vi "Connect to Slave.vi"(8 "error in (no error)":errorcluster, 11 "TCP master in":refnum<class "TCP.lvclass">) -> (0 "error out":errorcluster, 3 "TCP master out":refnum<class "TCP.lvclass">)   [LabVIEW 2021, in "TCP.lvclass"]
doc: "Opens a TCP connection to the address and port stored in the class."
uses:
  TCP.lvclass
  TCP.lvclass/TCP.ctl
  Transmission Data Unit/Transmission Data Unit.lvclass
  C:/my_projects/projects/Algorithms/Labview/21/Modbus_v121c/Network Protocol/MB/Modbus Master CR.lvclass
  C:/my_projects/projects/Algorithms/Labview/21/Modbus_v121c/Network Protocol/Network Master/Network Master.lvclass
  C:/my_projects/projects/Algorithms/Labview/21/Modbus_v121c/Network Protocol/Network Protocol.lvclass
  C:/my_projects/projects/Algorithms/Labview/21/Modbus_v121c/Network Protocol/ET7000/TCP/TCP.lvclass
  Network Master/Network Master.lvclass
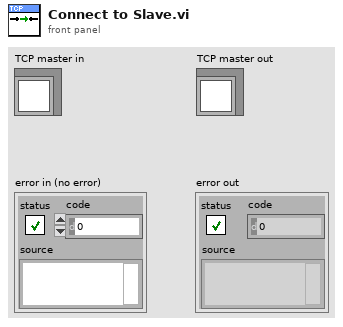
[diagram p1: front panel]
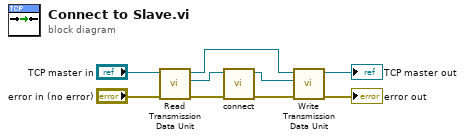
[diagram p0: block diagram]
diagram:
  n1 = call "Read Transmission Data Unit.vi"("error in (no error)"="error in (no error)", "Network Master in"="TCP master in") -> ("error out"=w4:errorcluster, "Transmission Data Unit"=w3:refnum<class "Transmission Data Unit.lvclass">, "Network Master out"=w9:refnum<class "TCP.lvclass">)  [unwired: 7 in]
  n2 = call-dynamic "connect.vi"("error in"=w4, "transmission data unit in"=w3) -> ("error out"=w2:errorcluster, "transmission data unit out"=w1:refnum<class "Transmission Data Unit.lvclass">)  [unwired: 8 in]
  n3 = call "Write Transmission Data Unit.vi"("error in (no error)"=w2, "Transmission Data Unit"=w1, "Network Master in"=w9) -> ("error out"=→"error out":errorcluster, "Network Master out"=→"TCP master out":refnum<class "TCP.lvclass">)  [unwired: 7 in]
